vi "ERROR.vi"() -> ()   [LabVIEW 2013]
panel:
  out "Result":dbl
  out "error out":errorcluster
  in  "error in (no error)":errorcluster
  in  "X":dbl
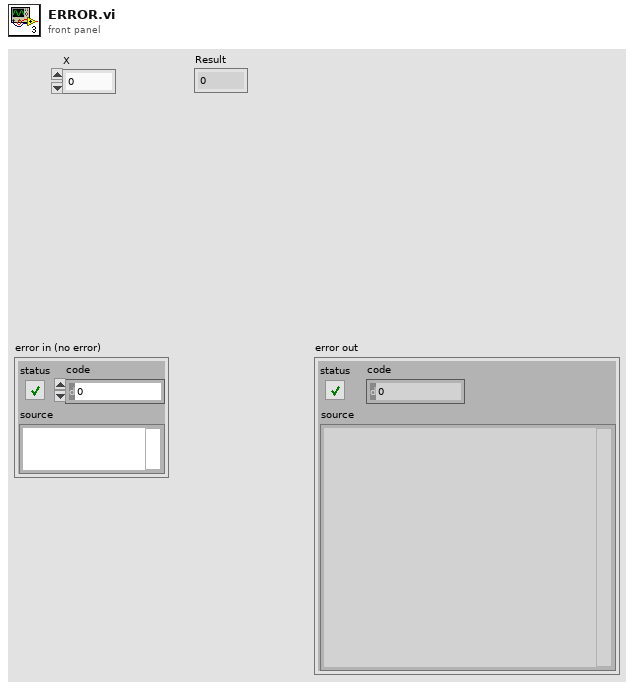
[diagram p1: front panel]
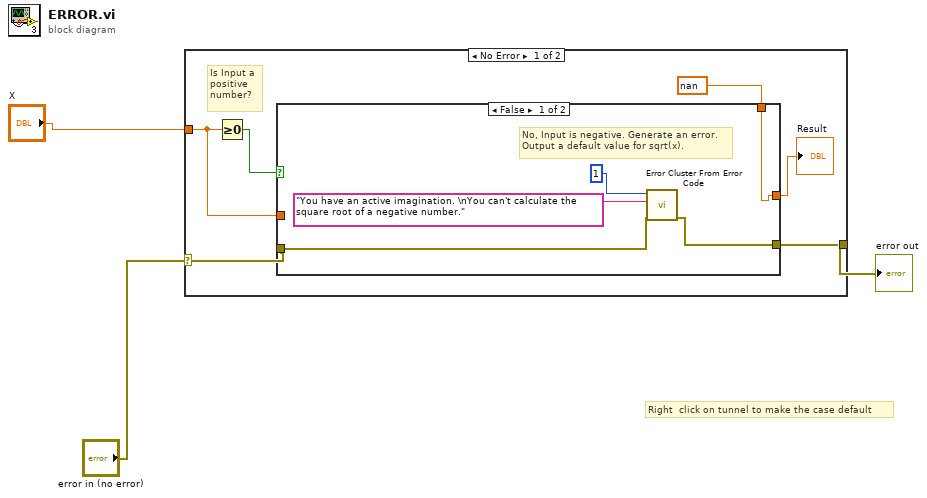
[diagram p0: block diagram]
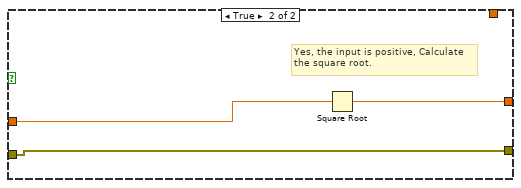
[diagram p2: hidden frame]
diagram:
  # "Right  click on tunnel to make the case default"
  n1 = case shown="No Error" "error in (no error)" {
    selector: "error in (no error)" -> [w7 w18]
    tunnel: "X" -> [w8 _]
    tunnel: [w6 w18] -> w1
    frame No Error {
      # "Is Input a \npositive \nnumber?"
      n2 = Greater Or Equal To 0?(x=w8) -> (x >= 0?=w9:bool)
      n3 = case shown="False" w9 {
        tunnel: w8 -> [_ w17]
        tunnel: [w10 w15] -> w5
        tunnel: w7 -> [w12 w16]
        tunnel: [w11 w16] -> w6
        tunnel: nan -> [w10 _]
        frame False {
          # "No, Input is negative. Generate an error.\nOutput a default value for sqrt(x)."
          n4 = call <vilib>:"Error Cluster From Error Code.vi"("error in (no error)"=w12, "error message (\"\")"="You have an active imagination. \nYou can't calculate the square root of a negative number." ("error message (\"\")"), "error code (0)"=1) -> ("error out"=w11:errorcluster)  [unwired: 6 in]
        }
        frame True {
          # "Yes, the input is positive, Calculate\nthe square root."
          n5 = Square Root(x=w17) -> (sqrt(x)=w15:dbl)
        }
      }
      "Result" <- w5
    }
    frame Error {
    }
  }
  "error out" <- w1
